vi "Lab Panel V6.00.vi"() -> ()   [LabVIEW 2017] (continued)
                      tunnel: w3847 -> [_ w3860 _ _]
                      tunnel: 0 -> [w3854 w3859 w3864 _]
                      tunnel: w3846 -> [_ _ w3865 _]
                      frame #0 {
                        n2193 = case shown="True" w3855 {
                          tunnel: w3854 -> [w3856 _]
                          frame False {
                            n2194 = local write "Er USB#0"(w3856) -> ()
                          }
                          frame True {
                            n2195 = local read "Er USB#0"() -> (w3858:dbl)
                            n2196 = Increment(x=w3858) -> (x+1=→"Er USB#0":dbl)
                          }
                        }
                      }
                      frame #1 {
                        n2197 = case shown="True" w3860 {
                          tunnel: w3859 -> [w3861 _]
                          frame False {
                            n2198 = local write "Er USB#1"(w3861) -> ()
                          }
                          frame True {
                            n2199 = local read "Er USB#1"() -> (w3863:dbl)
                            n2200 = Increment(x=w3863) -> (x+1=→"Er USB#1":dbl)
                          }
                        }
                      }
                      frame #2 {
                        n2201 = case shown="True" w3865 {
                          tunnel: w3864 -> [w3866 _]
                          frame False {
                            n2202 = local write "Er USB#2"(w3866) -> ()
                          }
                          frame True {
                            n2203 = local read "Er USB#2"() -> (w3868:dbl)
                            n2204 = Increment(x=w3868) -> (x+1=→"Er USB#2":dbl)
                          }
                        }
                      }
                      frame #3 {
                        w3874 = 10
                        n2205 = local read "Er USB#2"() -> (w3875:dbl)
                        n2206 = local read "Er USB#0"() -> (w3877:dbl)
                        n2207 = local read "Er USB#1"() -> (w3876:dbl)
                        n2208 = Greater Or Equal?(x=w3877, y=w3874) -> (x >= y?=w3872:bool)
                        n2209 = Greater Or Equal?(x=w3876, y=w3874) -> (x >= y?=w3871:bool)
                        n2210 = Greater Or Equal?(x=w3875, y=w3874) -> (x >= y?=w3870:bool)
                        n2211 = Or(x=w3872, y=w3871) -> (x .or. y?=w3873:bool)
                        n2212 = Or(x=w3873, y=w3870) -> (x .or. y?=→"Analog error":bool)
                      }
                    }
                  }
                  frame #1 {
                    # "display graph data on ADM page"
                    n2213 = local write "AI loop time"(w3878) -> ()
                    n2214 = local write "AI"(TRUE) -> ()
                    n2215 = Index Array(array=w3899, index=6) -> (element=→"LAB04-1 (GRAPH)":dynamicdata)
                    n2216 = Index Array(array=w3899, index=7) -> (element=→"LAB04-2 (GRAPH)":dynamicdata)
                    n2217 = Index Array(array=w3899, index=9) -> (element=→"LAB05-2 (GRAPH)":dynamicdata)
                    n2218 = Index Array(array=w3899, index=8) -> (element=→"LAB05-1 (GRAPH)":dynamicdata)
                    n2219 = Index Array(array=w3899, index=5) -> (element=→"LAB03-2 (GRAPH)":dynamicdata)
                    n2220 = Index Array(array=w3899, index=0) -> (element=→"LAB01-1 (GRAPH)":dynamicdata)
                    n2221 = Index Array(array=w3899, index=1) -> (element=→"LAB01-2 (GRAPH)":dynamicdata)
                    n2222 = Index Array(array=w3899, index=2) -> (element=→"LAB02-1 (GRAPH)":dynamicdata)
                    n2223 = Index Array(array=w3899, index=3) -> (element=→"LAB02-2 (GRAPH)":dynamicdata)
                    n2224 = Index Array(array=w3899, index=4) -> (element=→"LAB03-1 (GRAPH)":dynamicdata)
                  }
                  frame #2 {
                    n2225 = case shown="False" w3931 {
                      tunnel: [w3933 w3934] -> w3929
                      tunnel: w3930 -> [_ w3934]
                      frame False {
                        n2226 = local read "CAL LAB01"() -> (w3933:T15)
                      }
                      frame True {
                      }
                    }
                    n2227 = Unbundle By Name(w3932) -> ("OFF amps"=w3928:dbl, "VOLTS"=w3927:dbl, "PF"=w3926:dbl, "OFF amps"=w3925:dbl, "VOLTS"=w3924:dbl, "PF"=w3923:dbl)
                    n2228 = Unbundle By Name(w3929) -> ("1  (A) cal"=w3922:dbl, "1 (V) cal"=w3921:dbl, "1 (PF) cal"=w3920:dbl, "2 (A) cal"=w3919:dbl, "2 (V) cal"=w3918:dbl, "2 (PF) cal"=w3917:dbl)  [unwired: 4 out]
                    n2229 = Multiply(x=w3928, y=w3922) -> (x*y=w3912:dbl)
                    n2230 = Multiply(x=w3927, y=w3921) -> (x*y=w3911:dbl)
                    n2231 = Multiply(x=w3926, y=w3920) -> (x*y=w3906:dbl)
                    n2232 = Multiply(x=w3925, y=w3919) -> (x*y=w3909:dbl)
                    n2233 = Multiply(x=w3924, y=w3918) -> (x*y=w3908:dbl)
                    n2234 = Multiply(x=w3923, y=w3917) -> (x*y=w3902:dbl)
                    n2235 = local read "SIG LAB01-2"() -> (w3915:T2)
                    n2236 = call "Check for valid PF.vi"("PF In"=w3906, "VOLTS"=w3911, "Current"=w3912) -> ("PF Out"=w3904:dbl, "V Out"=w3905:dbl, "I Out"=w3910:dbl)  [unwired: 6 in]
                    n2237 = call "Check for valid PF.vi"("PF In"=w3902, "VOLTS"=w3908, "Current"=w3909) -> ("PF Out"=w3901:dbl, "V Out"=w3903:dbl, "I Out"=w3907:dbl)  [unwired: 6 in]
                    n2238 = local read "SIG LAB01-1"() -> (w3916:T2)
                    n2239 = Bundle By Name(cluster=w3916, "AMPS"=w3910, "VOLTS"=w3905, "PF"=w3904) -> (w3914:T2)
                    n2240 = Bundle By Name(cluster=w3915, "AMPS"=w3907, "VOLTS"=w3903, "PF"=w3901) -> (w3913:T2)
                    n2241 = global write "Global display 1.vi" "SIG LAB01-2"(w3913) -> ()
                    n2242 = global write "Global display 1.vi" "SIG LAB01-1"(w3914) -> ()
                    n2243 = local write "SIG LAB01-2"(w3913) -> ()
                    n2244 = local write "SIG LAB01-1"(w3914) -> ()
                  }
                  frame #3 {
                    n2245 = Unbundle By Name(w3966) -> ("OFF amps"=w3962:dbl, "VOLTS"=w3961:dbl, "PF"=w3960:dbl, "OFF amps"=w3959:dbl, "VOLTS"=w3958:dbl, "PF"=w3957:dbl)
                    n2246 = case shown="True" w3965 {
                      tunnel: [w3967 w3968] -> w3963
                      tunnel: w3964 -> [_ w3968]
                      frame False {
                        n2247 = local read "CAL LAB02"() -> (w3967:T16)
                      }
                      frame True {
                      }
                    }
                    n2248 = Unbundle By Name(w3963) -> ("1  (A) cal"=w3956:dbl, "1 (V) cal"=w3955:dbl, "1 (PF) cal"=w3954:dbl, "2 (A) cal"=w3953:dbl, "2 (V) cal"=w3952:dbl, "2 (PF) cal"=w3951:dbl)  [unwired: 4 out]
                    n2249 = Multiply(x=w3962, y=w3956) -> (x*y=w3946:dbl)
                    n2250 = Multiply(x=w3961, y=w3955) -> (x*y=w3945:dbl)
                    n2251 = Multiply(x=w3960, y=w3954) -> (x*y=w3938:dbl)
                    n2252 = Multiply(x=w3959, y=w3953) -> (x*y=w3943:dbl)
                    n2253 = Multiply(x=w3958, y=w3952) -> (x*y=w3942:dbl)
                    n2254 = Multiply(x=w3957, y=w3951) -> (x*y=w3937:dbl)
                    n2255 = local read "SIG LAB02-1"() -> (w3950:T2)
                    n2256 = local read "SIG LAB02-2"() -> (w3949:T2)
                    n2257 = call "Check for valid PF.vi"("PF In"=w3938, "VOLTS"=w3945, "Current"=w3946) -> ("PF Out"=w3940:dbl, "V Out"=w3939:dbl, "I Out"=w3944:dbl)  [unwired: 6 in]
                    n2258 = call "Check for valid PF.vi"("PF In"=w3937, "VOLTS"=w3942, "Current"=w3943) -> ("PF Out"=w3935:dbl, "V Out"=w3936:dbl, "I Out"=w3941:dbl)  [unwired: 6 in]
                    n2259 = Bundle By Name(cluster=w3950, "AMPS"=w3944, "VOLTS"=w3939, "PF"=w3940) -> (w3948:T2)
                    n2260 = Bundle By Name(cluster=w3949, "AMPS"=w3941, "VOLTS"=w3936, "PF"=w3935) -> (w3947:T2)
                    n2261 = global write "Global display 1.vi" "SIG LAB02-1"(w3948) -> ()
                    n2262 = local write "SIG LAB02-2"(w3947) -> ()
                    n2263 = global write "Global display 1.vi" "SIG LAB02-2"(w3947) -> ()
                    n2264 = local write "SIG LAB02-1"(w3948) -> ()
                  }
                  frame #4 {
                    n2265 = Unbundle By Name(w4000) -> ("OFF amps"=w3996:dbl, "VOLTS"=w3995:dbl, "PF"=w3994:dbl, "OFF amps"=w3993:dbl, "VOLTS"=w3992:dbl, "PF"=w3991:dbl)
                    n2266 = case shown="False" w3999 {
                      tunnel: [w4001 w4002] -> w3997
                      tunnel: w3998 -> [_ w4002]
                      frame False {
                        n2267 = local read "CAL LAB03"() -> (w4001:T15)
                      }
                      frame True {
                      }
                    }
                    n2268 = Unbundle By Name(w3997) -> ("1  (A) cal"=w3990:dbl, "1 (V) cal"=w3989:dbl, "1 (PF) cal"=w3988:dbl, "2 (A) cal"=w3987:dbl, "2 (V) cal"=w3986:dbl, "2 (PF) cal"=w3985:dbl)  [unwired: 4 out]
                    n2269 = Multiply(x=w3996, y=w3990) -> (x*y=w3980:dbl)
                    n2270 = Multiply(x=w3995, y=w3989) -> (x*y=w3979:dbl)
                    n2271 = Multiply(x=w3994, y=w3988) -> (x*y=w3974:dbl)
                    n2272 = Multiply(x=w3993, y=w3987) -> (x*y=w3977:dbl)
                    n2273 = Multiply(x=w3992, y=w3986) -> (x*y=w3976:dbl)
                    n2274 = Multiply(x=w3991, y=w3985) -> (x*y=w3973:dbl)
                    n2275 = local read "SIG LAB03-1"() -> (w3984:T2)
                    n2276 = local read "SIG LAB03-2"() -> (w3983:T2)
                    n2277 = call "Check for valid PF.vi"("PF In"=w3974, "VOLTS"=w3979, "Current"=w3980) -> ("PF Out"=w3969:dbl, "V Out"=w3970:dbl, "I Out"=w3978:dbl)  [unwired: 6 in]
                    n2278 = call "Check for valid PF.vi"("PF In"=w3973, "VOLTS"=w3976, "Current"=w3977) -> ("PF Out"=w3972:dbl, "V Out"=w3971:dbl, "I Out"=w3975:dbl)  [unwired: 6 in]
                    n2279 = Bundle By Name(cluster=w3984, "AMPS"=w3978, "VOLTS"=w3970, "PF"=w3969) -> (w3982:T2)
                    n2280 = Bundle By Name(cluster=w3983, "AMPS"=w3975, "VOLTS"=w3971, "PF"=w3972) -> (w3981:T2)
                    n2281 = global write "Global display 1.vi" "SIG LAB03-1"(w3982) -> ()
                    n2282 = global write "Global display 1.vi" "SIG LAB03-2"(w3981) -> ()
                    n2283 = local write "SIG LAB03-2"(w3981) -> ()
                    n2284 = local write "SIG LAB03-1"(w3982) -> ()
                  }
                  frame #5 {
                    n2285 = case shown="False" w4033 {
                      tunnel: [w4035 w4036] -> w4031
                      tunnel: w4032 -> [_ w4036]
                      frame False {
                        n2286 = local read "CAL LAB04"() -> (w4035:T15)
                      }
                      frame True {
                      }
                    }
                    n2287 = Unbundle By Name(w4034) -> ("OFF amps"=w4030:dbl, "VOLTS"=w4029:dbl, "PF"=w4028:dbl, "OFF amps"=w4027:dbl, "VOLTS"=w4026:dbl, "PF"=w4025:dbl)
                    n2288 = Unbundle By Name(w4031) -> ("1  (A) cal"=w4024:dbl, "1 (V) cal"=w4023:dbl, "1 (PF) cal"=w4022:dbl, "2 (A) cal"=w4021:dbl, "2 (V) cal"=w4020:dbl, "2 (PF) cal"=w4019:dbl)  [unwired: 4 out]
                    n2289 = Multiply(x=w4030, y=w4024) -> (x*y=w4014:dbl)
                    n2290 = Multiply(x=w4029, y=w4023) -> (x*y=w4013:dbl)
                    n2291 = Multiply(x=w4028, y=w4022) -> (x*y=w4004:dbl)
                    n2292 = Multiply(x=w4027, y=w4021) -> (x*y=w4011:dbl)
                    n2293 = Multiply(x=w4026, y=w4020) -> (x*y=w4010:dbl)
                    n2294 = Multiply(x=w4025, y=w4019) -> (x*y=w4003:dbl)
                    n2295 = local read "SIG LAB04-1"() -> (w4018:T2)
                    n2296 = local read "SIG LAB04-2"() -> (w4017:T2)
                    n2297 = call "Check for valid PF.vi"("PF In"=w4004, "VOLTS"=w4013, "Current"=w4014) -> ("PF Out"=w4007:dbl, "V Out"=w4008:dbl, "I Out"=w4012:dbl)  [unwired: 6 in]
                    n2298 = call "Check for valid PF.vi"("PF In"=w4003, "VOLTS"=w4010, "Current"=w4011) -> ("PF Out"=w4005:dbl, "V Out"=w4006:dbl, "I Out"=w4009:dbl)  [unwired: 6 in]
                    n2299 = Bundle By Name(cluster=w4018, "AMPS"=w4012, "VOLTS"=w4008, "PF"=w4007) -> (w4016:T2)
                    n2300 = Bundle By Name(cluster=w4017, "AMPS"=w4009, "VOLTS"=w4006, "PF"=w4005) -> (w4015:T2)
                    n2301 = global write "Global display 1.vi" "SIG LAB04-2"(w4015) -> ()
                    n2302 = global write "Global display 1.vi" "SIG LAB04-1"(w4016) -> ()
                    n2303 = local write "SIG LAB04-2"(w4015) -> ()
                    n2304 = local write "SIG LAB04-1"(w4016) -> ()
                  }
                  frame #6 {
                    n2305 = Unbundle By Name(w4068) -> ("OFF amps"=w4064:dbl, "VOLTS"=w4051:dbl, "PF"=w4063:dbl, "OFF amps"=w4062:dbl, "VOLTS"=w4061:dbl, "PF"=w4060:dbl)
                    n2306 = case shown="False" w4067 {
                      tunnel: [w4069 w4070] -> w4065
                      tunnel: w4066 -> [_ w4070]
                      frame False {
                        n2307 = local read "CAL LAB05"() -> (w4069:T15)
                      }
                      frame True {
                      }
                    }
                    n2308 = Unbundle By Name(w4065) -> ("1  (A) cal"=w4059:dbl, "1 (V) cal"=w4058:dbl, "1 (PF) cal"=w4057:dbl, "2 (A) cal"=w4056:dbl, "2 (V) cal"=w4055:dbl, "2 (PF) cal"=w4054:dbl)  [unwired: 4 out]
                    n2309 = Multiply(x=w4064, y=w4059) -> (x*y=w4048:dbl)
                    n2310 = Multiply(x=w4051, y=w4058) -> (x*y=w4047:dbl)
                    n2311 = Multiply(x=w4063, y=w4057) -> (x*y=w4042:dbl)
                    n2312 = Multiply(x=w4062, y=w4056) -> (x*y=w4045:dbl)
                    n2313 = Multiply(x=w4061, y=w4055) -> (x*y=w4044:dbl)
                    n2314 = Multiply(x=w4060, y=w4054) -> (x*y=w4039:dbl)
                    n2315 = local read "SIG LAB05-1"() -> (w4053:T2)
                    n2316 = local read "SIG LAB05-2"() -> (w4052:T2)
                    n2317 = call "Check for valid PF.vi"("PF In"=w4039, "VOLTS"=w4044, "Current"=w4045) -> ("PF Out"=w4038:dbl, "V Out"=w4037:dbl, "I Out"=w4043:dbl)  [unwired: 6 in]
                    n2318 = call "Check for valid PF.vi"("PF In"=w4042, "VOLTS"=w4047, "Current"=w4048) -> ("PF Out"=w4041:dbl, "V Out"=w4040:dbl, "I Out"=w4046:dbl)  [unwired: 6 in]
                    n2319 = Bundle By Name(cluster=w4053, "AMPS"=w4046, "VOLTS"=w4040, "PF"=w4041) -> (w4050:T2)
                    n2320 = Bundle By Name(cluster=w4052, "AMPS"=w4043, "VOLTS"=w4037, "PF"=w4038) -> (w4049:T2)
                    n2321 = global write "Global display 1.vi" "SIG LAB05-1"(w4050) -> ()
                    n2322 = global write "Global display 1.vi" "SIG LAB05-2"(w4049) -> ()
                    n2323 = local write "SIG LAB05-2"(w4049) -> ()
                    n2324 = local write "SIG LAB05-1"(w4050) -> ()
                  }
                  frame #7 {
                    n2325 = case shown="False" w4071 {
                      tunnel: w4073 -> [w4078 _]
                      tunnel: w4072 -> [w4077 _]
                      frame False {
                        # "update ambient referance temperature"
                        n2326 = case shown="False" w4078 {
                          tunnel: [w4080 100.0] -> w4079
                          frame False {
                            n2327 = local read "TEMP REF cal"() -> (w4080:dbl)
                          }
                          frame True {
                          }
                        }
                        n2328 = disable-structure shown="Disabled" {
                          frame Disabled {
                            n2329 = local read "Temp read loop"() -> ()  [unwired: 1 out]
                          }
                          frame Enabled {
                          }
                        }
                        n2330 = Multiply(x=w4079, y=w4077) -> (x*y=w4076:dbl)
                        n2331 = Subtract(x=w4076, y=272) -> (x-y=w4074:dbl)
                        "Amb Temp" <- w4074
                        n2332 = local write "Ref deg C"(w4074) -> ()
                        "deg C (volts)" <- w4077
                      }
                      frame True {
                      }
                    }
                  }
                }
              }
            }
          }
          frame #14 {
            # "save test data to file during testing"
            n2333 = local read "on loops"() -> (w4101:dbl)
            n2334 = Get Date/Time In Seconds() -> (seconds since 1Jan1904=w4082:timestamp)
            "File Time Stamp" <- w4082
            n2335 = local read "jig cycle"() -> (w4098:dbl)
            n2336 = Format Date/Time String(time format string (%c)="%H:%M%:%S", seconds (now)=w4082) -> (date/time string=w4086:string)  [unwired: 1 in]
            n2337 = Add(x=w4101, y=4) -> (x+y=w4099:dbl)
            n2338 = Build Array(w4086) -> (w4085:string[])
            n2339 = Equal?(x=w4098, y=3) -> (x = y?=w4084:bool)
            n2340 = Equal?(x=w4098, y=w4099) -> (x = y?=w4083:bool)
            n2341 = stacked-sequence {
              tunnel: w4097 -> [w4107 _ _ _ _ _ _ _ _ _]
              tunnel: w4096 -> [_ w4183 _ _ _ _ _ _ _ _]
              tunnel: w4095 -> [_ _ w4263 _ _ _ _ _ _ _]
              tunnel: w4094 -> [_ _ _ w4343 _ _ _ _ _ _]
              tunnel: w4093 -> [_ _ _ _ w4423 _ _ _ _ _]
              tunnel: w4092 -> [_ _ _ _ _ w4503 _ _ _ _]
              tunnel: w4091 -> [_ _ _ _ _ _ w4583 _ _ _]
              tunnel: w4090 -> [_ _ _ _ _ _ _ w4663 _ _]
              tunnel: w4089 -> [_ _ _ _ _ _ _ _ w4743 _]
              tunnel: w4088 -> [_ _ _ _ _ _ _ _ _ w4823]
              tunnel: w4085 -> [w4106 w4187 w4267 w4347 w4427 w4507 w4587 w4667 w4747 w4827]
              tunnel: w4084 -> [w4105 w4186 w4266 w4346 w4426 w4506 w4586 w4666 w4746 w4826]
              tunnel: w4083 -> [w4104 w4185 w4265 w4345 w4425 w4505 w4585 w4665 w4745 w4825]
              tunnel: w4082 -> [w4103 w4184 w4264 w4344 w4424 w4504 w4584 w4664 w4744 w4824]
              frame #0 {
                n2342 = case shown="True" w4107 {
                  tunnel: w4106 -> [_ w4112]
                  tunnel: w4105 -> [_ w4111]
                  tunnel: w4104 -> [_ w4109]
                  tunnel: w4103 -> [_ w4108]
                  frame False {
                  }
                  frame True {
                    n2343 = local read "SIG LAB01-1"() -> (w4114:T2)
                    n2344 = local read "ON L01-1"() -> (w4110:cluster{"amps":dbl, "volts":dbl, "pf":dbl})
                    n2345 = local read "DISP LAB01-1"() -> (w4113:T4)
                    n2346 = Unbundle(w4114) -> ("AMPS"=w4120:dbl, "VOLTS"=w4118:dbl, "PF"=w4117:dbl, "Tmp Live"=w4116:dbl, "Tmp Neut"=w4119:dbl)
                    n2347 = Unbundle(w4113) -> ("CYCLE"=w4115:dbl)  [unwired: 2 out]
                    n2348 = stacked-sequence {
                      tunnel: w4120 -> [w4124 w4143]
                      tunnel: w4119 -> [_ w4142]
                      tunnel: w4118 -> [w4123 w4141]
                      tunnel: w4117 -> [w4122 w4140]
                      tunnel: w4116 -> [_ w4139]
                      tunnel: w4115 -> [_ w4138]
                      tunnel: w4112 -> [_ w4137]
                      tunnel: w4111 -> [w4125 _]
                      tunnel: w4110 -> [w4121 w4135]
                      tunnel: w4109 -> [_ w4136]
                      tunnel: w4108 -> [_ w4131]
                      frame #0 {
                        n2349 = case shown="True" w4125 {
                          tunnel: w4124 -> [_ w4130]
                          tunnel: w4123 -> [_ w4129]
                          tunnel: w4122 -> [_ w4128]
                          tunnel: w4121 -> [_ w4126]
                          frame False {
                          }
                          frame True {
                            n2350 = Bundle(cluster=w4126, "amps"=w4130, "volts"=w4129, "pf"=w4128) -> (w4127:cluster{"amps":dbl, "volts":dbl, "pf":dbl})
                            n2351 = local write "ON L01-1"(w4127) -> ()
                          }
                        }
                      }
                      frame #1 {
                        n2352 = Unbundle(w4135) -> ("amps"=w4134:dbl, "volts"=w4133:dbl, "pf"=w4132:dbl)
                        n2353 = case shown="True" w4136 {
                          tunnel: w4143 -> [_ w4144]
                          tunnel: w4142 -> [_ w4182]
                          tunnel: w4141 -> [_ _]
                          tunnel: w4140 -> [_ _]
                          tunnel: w4139 -> [_ w4181]
                          tunnel: w4138 -> [_ w4180]
                          tunnel: w4137 -> [_ w4148]
                          tunnel: w4134 -> [_ w4145]
                          tunnel: w4133 -> [_ w4177]
                          tunnel: w4132 -> [_ w4176]
                          tunnel: w4131 -> [_ w4146]
                          frame False {
                          }
                          frame True {
                            n2354 = local read "TDMS LAB01-1"() -> (w4179:refnum<k34>)
                            n2355 = Build Array(w4177) -> (w4173:dbl[])
                            n2356 = Build Array(w4176) -> (w4172:dbl[])
                            n2357 = Build Array(w4181) -> (w4171:dbl[])
                            n2358 = Build Array(w4182) -> (w4170:dbl[])
                            n2359 = Build Array(w4145) -> (w4175:dbl[])
                            n2360 = Build Array(w4144) -> (w4174:dbl[])
                            n2361 = Build Array(w4180) -> (w4169:dbl[])
                            n2362 = Build Array("AMPS ON", "AMPS OFF", "VOLTS", "PF", "TEMP Live", "TEMP Neut", "CYCLE") -> (w4153:string[])
                            n2363 = Bundle By Name("Y"=w4175, "t0"=w4146) -> (w4168:waveform(dbl))  [unwired: 1 in]
                            n2364 = Bundle By Name("Y"=w4174, "t0"=w4146) -> (w4167:waveform(dbl))  [unwired: 1 in]
                            n2365 = Bundle By Name("Y"=w4173, "t0"=w4146) -> (w4166:waveform(dbl))  [unwired: 1 in]
                            n2366 = Bundle By Name("Y"=w4172, "t0"=w4146) -> (w4165:waveform(dbl))  [unwired: 1 in]
                            n2367 = Bundle By Name("Y"=w4171, "t0"=w4146) -> (w4164:waveform(dbl))  [unwired: 1 in]
                            n2368 = Bundle By Name("Y"=w4170, "t0"=w4146) -> (w4163:waveform(dbl))  [unwired: 1 in]
                            n2369 = Bundle By Name("Y"=w4169, "t0"=w4146) -> (w4162:waveform(dbl))  [unwired: 1 in]
                            n2370 = Build Array(w4168, w4167, w4166, w4165, w4164, w4163, w4162) -> (w4161:waveform(dbl)[])
                            n2371 = TDMS Write(0:w4179, 5:"TEST VALUES", 7:w4153, 9:w4161) -> (4:w4152:refnum<k34>, 6:w4151:string, 15:w4150:errorcluster)  [unwired: 2 in, 1 out]
                            n2372 = TDMS Write(0:w4152, 5:w4151, 7:"TIME", 9:w4148, 11:w4150) -> (15:w4147:errorcluster)  [unwired: 1 in, 3 out]
                            n2373 = local write "data file error"(w4147) -> ()
                          }
                        }
                      }
                    }
                  }
                }
              }
              frame #1 {
                n2374 = case shown="True" w4183 {
                  tunnel: w4187 -> [_ w4192]
                  tunnel: w4186 -> [_ w4191]
                  tunnel: w4185 -> [_ w4189]
                  tunnel: w4184 -> [_ w4188]
                  frame False {
                  }
                  frame True {
                    n2375 = local read "DISP LAB01-2"() -> (w4193:T4)
                    n2376 = local read "SIG LAB01-2"() -> (w4194:T2)
                    n2377 = local read "ON L01-2"() -> (w4190:cluster{"amps":dbl, "volts":dbl, "pf":dbl})
                    n2378 = Unbundle(w4194) -> ("AMPS"=w4200:dbl, "VOLTS"=w4198:dbl, "PF"=w4197:dbl, "Tmp Live"=w4196:dbl, "Tmp Neut"=w4199:dbl)
                    n2379 = Unbundle(w4193) -> ("CYCLE"=w4195:dbl)  [unwired: 2 out]
                    n2380 = stacked-sequence {
                      tunnel: w4200 -> [w4204 w4223]
                      tunnel: w4199 -> [_ w4222]
                      tunnel: w4198 -> [w4203 w4221]
                      tunnel: w4197 -> [w4202 w4220]
                      tunnel: w4196 -> [_ w4219]
                      tunnel: w4195 -> [_ w4218]
                      tunnel: w4192 -> [_ w4217]
                      tunnel: w4191 -> [w4205 _]
                      tunnel: w4190 -> [w4201 w4215]
                      tunnel: w4189 -> [_ w4216]
                      tunnel: w4188 -> [_ w4211]
                      frame #0 {
                        n2381 = case shown="True" w4205 {
                          tunnel: w4204 -> [_ w4210]
                          tunnel: w4203 -> [_ w4209]
                          tunnel: w4202 -> [_ w4208]
                          tunnel: w4201 -> [_ w4206]
                          frame False {
                          }
                          frame True {
                            n2382 = Bundle(cluster=w4206, "amps"=w4210, "volts"=w4209, "pf"=w4208) -> (w4207:cluster{"amps":dbl, "volts":dbl, "pf":dbl})
                            n2383 = local write "ON L01-2"(w4207) -> ()
                          }
                        }
                      }
                      frame #1 {
                        n2384 = Unbundle(w4215) -> ("amps"=w4214:dbl, "volts"=w4213:dbl, "pf"=w4212:dbl)
                        n2385 = case shown="True" w4216 {
                          tunnel: w4223 -> [_ w4255]
                          tunnel: w4222 -> [_ w4262]
                          tunnel: w4221 -> [_ _]
                          tunnel: w4220 -> [_ _]
                          tunnel: w4219 -> [_ w4261]
                          tunnel: w4218 -> [_ w4260]
                          tunnel: w4217 -> [_ w4225]
                          tunnel: w4214 -> [_ w4257]
                          tunnel: w4213 -> [_ w4256]
                          tunnel: w4212 -> [_ w4254]
                          tunnel: w4211 -> [_ w4246]
                          frame False {
                          }
                          frame True {
                            n2386 = local read "TDMS LAB01-2"() -> (w4259:refnum<k34>)
                            n2387 = Build Array(w4256) -> (w4251:dbl[])
                            n2388 = Build Array(w4254) -> (w4250:dbl[])
                            n2389 = Build Array(w4261) -> (w4249:dbl[])
                            n2390 = Build Array(w4262) -> (w4248:dbl[])
                            n2391 = Build Array(w4257) -> (w4253:dbl[])
                            n2392 = Build Array(w4255) -> (w4252:dbl[])
                            n2393 = Build Array(w4260) -> (w4247:dbl[])
                            n2394 = Build Array("AMPS ON", "AMPS OFF", "VOLTS", "PF", "TEMP Live", "TEMP Neut", "CYCLE") -> (w4230:string[])
                            n2395 = Bundle By Name("Y"=w4253, "t0"=w4246) -> (w4245:waveform(dbl))  [unwired: 1 in]
                            n2396 = Bundle By Name("Y"=w4252, "t0"=w4246) -> (w4244:waveform(dbl))  [unwired: 1 in]
                            n2397 = Bundle By Name("Y"=w4251, "t0"=w4246) -> (w4243:waveform(dbl))  [unwired: 1 in]
                            n2398 = Bundle By Name("Y"=w4250, "t0"=w4246) -> (w4242:waveform(dbl))  [unwired: 1 in]
                            n2399 = Bundle By Name("Y"=w4249, "t0"=w4246) -> (w4241:waveform(dbl))  [unwired: 1 in]
                            n2400 = Bundle By Name("Y"=w4248, "t0"=w4246) -> (w4240:waveform(dbl))  [unwired: 1 in]
                            n2401 = Bundle By Name("Y"=w4247, "t0"=w4246) -> (w4239:waveform(dbl))  [unwired: 1 in]
                            n2402 = Build Array(w4245, w4244, w4243, w4242, w4241, w4240, w4239) -> (w4238:waveform(dbl)[])
                            n2403 = TDMS Write(0:w4259, 5:"TEST VALUES", 7:w4230, 9:w4238) -> (4:w4229:refnum<k34>, 6:w4228:string, 15:w4227:errorcluster)  [unwired: 2 in, 1 out]
                            n2404 = TDMS Write(0:w4229, 5:w4228, 7:"TIME", 9:w4225, 11:w4227) -> (15:w4224:errorcluster)  [unwired: 1 in, 3 out]
                            n2405 = local write "data file error"(w4224) -> ()
                          }
                        }
                      }
                    }
                  }
                }
              }
              frame #2 {
                n2406 = case shown="True" w4263 {
                  tunnel: w4267 -> [_ w4272]
                  tunnel: w4266 -> [_ w4271]
                  tunnel: w4265 -> [_ w4269]
                  tunnel: w4264 -> [_ w4268]
                  frame False {
                  }
                  frame True {
                    n2407 = local read "DISP LAB02-1"() -> (w4273:T4)
                    n2408 = local read "SIG LAB02-1"() -> (w4274:T2)
                    n2409 = local read "ON L02-1"() -> (w4270:cluster{"amps":dbl, "volts":dbl, "pf":dbl})
                    n2410 = Unbundle(w4274) -> ("AMPS"=w4280:dbl, "VOLTS"=w4278:dbl, "PF"=w4277:dbl, "Tmp Live"=w4276:dbl, "Tmp Neut"=w4279:dbl)
                    n2411 = Unbundle(w4273) -> ("CYCLE"=w4275:dbl)  [unwired: 2 out]
                    n2412 = stacked-sequence {
                      tunnel: w4280 -> [w4284 w4303]
                      tunnel: w4279 -> [_ w4302]
                      tunnel: w4278 -> [w4283 w4301]
                      tunnel: w4277 -> [w4282 w4300]
                      tunnel: w4276 -> [_ w4299]
                      tunnel: w4275 -> [_ w4298]
                      tunnel: w4272 -> [_ w4297]
                      tunnel: w4271 -> [w4285 _]
                      tunnel: w4270 -> [w4281 w4295]
                      tunnel: w4269 -> [_ w4296]
                      tunnel: w4268 -> [_ w4291]
                      frame #0 {
                        n2413 = case shown="True" w4285 {
                          tunnel: w4284 -> [_ w4290]
                          tunnel: w4283 -> [_ w4289]
                          tunnel: w4282 -> [_ w4288]
                          tunnel: w4281 -> [_ w4286]
                          frame False {
                          }
                          frame True {
                            n2414 = Bundle(cluster=w4286, "amps"=w4290, "volts"=w4289, "pf"=w4288) -> (w4287:cluster{"amps":dbl, "volts":dbl, "pf":dbl})
                            n2415 = local write "ON L02-1"(w4287) -> ()
                          }
                        }
                      }
                      frame #1 {
                        n2416 = Unbundle(w4295) -> ("amps"=w4294:dbl, "volts"=w4293:dbl, "pf"=w4292:dbl)
                        n2417 = case shown="True" w4296 {
                          tunnel: w4303 -> [_ w4335]
                          tunnel: w4302 -> [_ w4342]
                          tunnel: w4301 -> [_ _]
                          tunnel: w4300 -> [_ _]
                          tunnel: w4299 -> [_ w4341]
                          tunnel: w4298 -> [_ w4340]
                          tunnel: w4297 -> [_ w4305]
                          tunnel: w4294 -> [_ w4337]
                          tunnel: w4293 -> [_ w4336]
                          tunnel: w4292 -> [_ w4334]
                          tunnel: w4291 -> [_ w4326]
                          frame False {
                          }
                          frame True {
                            n2418 = local read "TDMS LAB02-1"() -> (w4339:refnum<k34>)
                            n2419 = Build Array(w4336) -> (w4331:dbl[])
                            n2420 = Build Array(w4334) -> (w4330:dbl[])
                            n2421 = Build Array(w4341) -> (w4329:dbl[])
                            n2422 = Build Array(w4342) -> (w4328:dbl[])
                            n2423 = Build Array(w4337) -> (w4333:dbl[])
                            n2424 = Build Array(w4335) -> (w4332:dbl[])
                            n2425 = Build Array(w4340) -> (w4327:dbl[])
                            n2426 = Build Array("AMPS ON", "AMPS OFF", "VOLTS", "PF", "TEMP Live", "TEMP Neut", "CYCLE") -> (w4310:string[])
                            n2427 = Bundle By Name("Y"=w4333, "t0"=w4326) -> (w4325:waveform(dbl))  [unwired: 1 in]
                            n2428 = Bundle By Name("Y"=w4332, "t0"=w4326) -> (w4324:waveform(dbl))  [unwired: 1 in]
                            n2429 = Bundle By Name("Y"=w4331, "t0"=w4326) -> (w4323:waveform(dbl))  [unwired: 1 in]
                            n2430 = Bundle By Name("Y"=w4330, "t0"=w4326) -> (w4322:waveform(dbl))  [unwired: 1 in]
                            n2431 = Bundle By Name("Y"=w4329, "t0"=w4326) -> (w4321:waveform(dbl))  [unwired: 1 in]
                            n2432 = Bundle By Name("Y"=w4328, "t0"=w4326) -> (w4320:waveform(dbl))  [unwired: 1 in]
                            n2433 = Bundle By Name("Y"=w4327, "t0"=w4326) -> (w4319:waveform(dbl))  [unwired: 1 in]
                            n2434 = Build Array(w4325, w4324, w4323, w4322, w4321, w4320, w4319) -> (w4318:waveform(dbl)[])
                            n2435 = TDMS Write(0:w4339, 5:"TEST VALUES", 7:w4310, 9:w4318) -> (4:w4309:refnum<k34>, 6:w4308:string, 15:w4307:errorcluster)  [unwired: 2 in, 1 out]
                            n2436 = TDMS Write(0:w4309, 5:w4308, 7:"TIME", 9:w4305, 11:w4307) -> (15:w4304:errorcluster)  [unwired: 1 in, 3 out]
                            n2437 = local write "data file error"(w4304) -> ()
                          }
                        }
                      }
                    }
                  }
                }
              }
              frame #3 {
                n2438 = case shown="True" w4343 {
                  tunnel: w4347 -> [_ w4352]
                  tunnel: w4346 -> [_ w4351]
                  tunnel: w4345 -> [_ w4349]
                  tunnel: w4344 -> [_ w4348]
                  frame False {
                  }
                  frame True {
                    n2439 = local read "DISP LAB02-2"() -> (w4353:T4)
                    n2440 = local read "SIG LAB02-2"() -> (w4354:T2)
                    n2441 = local read "ON L02-2"() -> (w4350:cluster{"amps":dbl, "volts":dbl, "pf":dbl})
                    n2442 = Unbundle(w4354) -> ("AMPS"=w4360:dbl, "VOLTS"=w4358:dbl, "PF"=w4357:dbl, "Tmp Live"=w4356:dbl, "Tmp Neut"=w4359:dbl)
                    n2443 = Unbundle(w4353) -> ("CYCLE"=w4355:dbl)  [unwired: 2 out]
                    n2444 = stacked-sequence {
                      tunnel: w4360 -> [w4364 w4383]
                      tunnel: w4359 -> [_ w4382]
                      tunnel: w4358 -> [w4363 w4381]
                      tunnel: w4357 -> [w4362 w4380]
                      tunnel: w4356 -> [_ w4379]
                      tunnel: w4355 -> [_ w4378]
                      tunnel: w4352 -> [_ w4377]
                      tunnel: w4351 -> [w4365 _]
                      tunnel: w4350 -> [w4361 w4375]
                      tunnel: w4349 -> [_ w4376]
                      tunnel: w4348 -> [_ w4371]
                      frame #0 {
                        n2445 = case shown="True" w4365 {
                          tunnel: w4364 -> [_ w4370]
                          tunnel: w4363 -> [_ w4369]
                          tunnel: w4362 -> [_ w4368]
                          tunnel: w4361 -> [_ w4366]
                          frame False {
                          }
                          frame True {
                            n2446 = Bundle(cluster=w4366, "amps"=w4370, "volts"=w4369, "pf"=w4368) -> (w4367:cluster{"amps":dbl, "volts":dbl, "pf":dbl})
                            n2447 = local write "ON L02-2"(w4367) -> ()
                          }
                        }
                      }
                      frame #1 {
                        n2448 = Unbundle(w4375) -> ("amps"=w4374:dbl, "volts"=w4373:dbl, "pf"=w4372:dbl)
                        n2449 = case shown="True" w4376 {
                          tunnel: w4383 -> [_ w4415]
                          tunnel: w4382 -> [_ w4422]
                          tunnel: w4381 -> [_ _]
                          tunnel: w4380 -> [_ _]
                          tunnel: w4379 -> [_ w4421]
                          tunnel: w4378 -> [_ w4420]
                          tunnel: w4377 -> [_ w4385]
                          tunnel: w4374 -> [_ w4417]
                          tunnel: w4373 -> [_ w4416]
                          tunnel: w4372 -> [_ w4414]
                          tunnel: w4371 -> [_ w4406]
                          frame False {
                          }
                          frame True {
                            n2450 = local read "TDMS LAB02-2"() -> (w4419:refnum<k34>)
                            n2451 = Build Array(w4416) -> (w4411:dbl[])
                            n2452 = Build Array(w4414) -> (w4410:dbl[])
                            n2453 = Build Array(w4421) -> (w4409:dbl[])
                            n2454 = Build Array(w4422) -> (w4408:dbl[])
                            n2455 = Build Array(w4417) -> (w4413:dbl[])
                            n2456 = Build Array(w4415) -> (w4412:dbl[])
                            n2457 = Build Array(w4420) -> (w4407:dbl[])
                            n2458 = Build Array("AMPS ON", "AMPS OFF", "VOLTS", "PF", "TEMP Live", "TEMP Neut", "CYCLE") -> (w4390:string[])
                            n2459 = Bundle By Name("Y"=w4413, "t0"=w4406) -> (w4405:waveform(dbl))  [unwired: 1 in]
                            n2460 = Bundle By Name("Y"=w4412, "t0"=w4406) -> (w4404:waveform(dbl))  [unwired: 1 in]
                            n2461 = Bundle By Name("Y"=w4411, "t0"=w4406) -> (w4403:waveform(dbl))  [unwired: 1 in]
                            n2462 = Bundle By Name("Y"=w4410, "t0"=w4406) -> (w4402:waveform(dbl))  [unwired: 1 in]
                            n2463 = Bundle By Name("Y"=w4409, "t0"=w4406) -> (w4401:waveform(dbl))  [unwired: 1 in]
                            n2464 = Bundle By Name("Y"=w4408, "t0"=w4406) -> (w4400:waveform(dbl))  [unwired: 1 in]
                            n2465 = Bundle By Name("Y"=w4407, "t0"=w4406) -> (w4399:waveform(dbl))  [unwired: 1 in]
                            n2466 = Build Array(w4405, w4404, w4403, w4402, w4401, w4400, w4399) -> (w4398:waveform(dbl)[])
                            n2467 = TDMS Write(0:w4419, 5:"TEST VALUES", 7:w4390, 9:w4398) -> (4:w4389:refnum<k34>, 6:w4388:string, 15:w4387:errorcluster)  [unwired: 2 in, 1 out]
                            n2468 = TDMS Write(0:w4389, 5:w4388, 7:"TIME", 9:w4385, 11:w4387) -> (15:w4384:errorcluster)  [unwired: 1 in, 3 out]
                            n2469 = local write "data file error"(w4384) -> ()
                          }
                        }
                      }
                    }
                  }
                }
              }
              frame #4 {
                n2470 = case shown="True" w4423 {
                  tunnel: w4427 -> [_ w4432]
                  tunnel: w4426 -> [_ w4431]
                  tunnel: w4425 -> [_ w4429]
                  tunnel: w4424 -> [_ w4428]
                  frame False {
                  }
                  frame True {
                    n2471 = local read "DISP LAB03-1"() -> (w4433:T4)
                    n2472 = local read "SIG LAB03-1"() -> (w4434:T2)
                    n2473 = local read "ON L03-1"() -> (w4430:cluster{"amps":dbl, "volts":dbl, "pf":dbl})
                    n2474 = Unbundle(w4434) -> ("AMPS"=w4440:dbl, "VOLTS"=w4438:dbl, "PF"=w4437:dbl, "Tmp Live"=w4436:dbl, "Tmp Neut"=w4439:dbl)
                    n2475 = Unbundle(w4433) -> ("CYCLE"=w4435:dbl)  [unwired: 2 out]
                    n2476 = stacked-sequence {
                      tunnel: w4440 -> [w4444 w4463]
                      tunnel: w4439 -> [_ w4462]
                      tunnel: w4438 -> [w4443 w4461]
                      tunnel: w4437 -> [w4442 w4460]
                      tunnel: w4436 -> [_ w4459]
                      tunnel: w4435 -> [_ w4458]
                      tunnel: w4432 -> [_ w4457]
                      tunnel: w4431 -> [w4445 _]
                      tunnel: w4430 -> [w4441 w4455]
                      tunnel: w4429 -> [_ w4456]
                      tunnel: w4428 -> [_ w4451]
                      frame #0 {
                        n2477 = case shown="True" w4445 {
                          tunnel: w4444 -> [_ w4450]
                          tunnel: w4443 -> [_ w4449]
                          tunnel: w4442 -> [_ w4448]
                          tunnel: w4441 -> [_ w4446]
                          frame False {
                          }
                          frame True {
                            n2478 = Bundle(cluster=w4446, "amps"=w4450, "volts"=w4449, "pf"=w4448) -> (w4447:cluster{"amps":dbl, "volts":dbl, "pf":dbl})
                            n2479 = local write "ON L03-1"(w4447) -> ()
                          }
                        }
                      }
                      frame #1 {
                        n2480 = Unbundle(w4455) -> ("amps"=w4454:dbl, "volts"=w4453:dbl, "pf"=w4452:dbl)
                        n2481 = case shown="True" w4456 {
                          tunnel: w4463 -> [_ w4495]
                          tunnel: w4462 -> [_ w4502]
                          tunnel: w4461 -> [_ _]
                          tunnel: w4460 -> [_ _]
                          tunnel: w4459 -> [_ w4501]
                          tunnel: w4458 -> [_ w4500]
                          tunnel: w4457 -> [_ w4465]
                          tunnel: w4454 -> [_ w4497]
                          tunnel: w4453 -> [_ w4496]
                          tunnel: w4452 -> [_ w4494]
                          tunnel: w4451 -> [_ w4486]
                          frame False {
                          }
                          frame True {
                            n2482 = local read "TDMS LAB03-1"() -> (w4499:refnum<k34>)
                            n2483 = Build Array(w4496) -> (w4491:dbl[])
                            n2484 = Build Array(w4494) -> (w4490:dbl[])
                            n2485 = Build Array(w4501) -> (w4489:dbl[])
                            n2486 = Build Array(w4502) -> (w4488:dbl[])
                            n2487 = Build Array(w4497) -> (w4493:dbl[])
                            n2488 = Build Array(w4495) -> (w4492:dbl[])
                            n2489 = Build Array(w4500) -> (w4487:dbl[])
                            n2490 = Build Array("AMPS ON", "AMPS OFF", "VOLTS", "PF", "TEMP Live", "TEMP Neut", "CYCLE") -> (w4470:string[])
                            n2491 = Bundle By Name("Y"=w4493, "t0"=w4486) -> (w4485:waveform(dbl))  [unwired: 1 in]
                            n2492 = Bundle By Name("Y"=w4492, "t0"=w4486) -> (w4484:waveform(dbl))  [unwired: 1 in]
                            n2493 = Bundle By Name("Y"=w4491, "t0"=w4486) -> (w4483:waveform(dbl))  [unwired: 1 in]
                            n2494 = Bundle By Name("Y"=w4490, "t0"=w4486) -> (w4482:waveform(dbl))  [unwired: 1 in]
                            n2495 = Bundle By Name("Y"=w4489, "t0"=w4486) -> (w4481:waveform(dbl))  [unwired: 1 in]
                            n2496 = Bundle By Name("Y"=w4488, "t0"=w4486) -> (w4480:waveform(dbl))  [unwired: 1 in]
                            n2497 = Bundle By Name("Y"=w4487, "t0"=w4486) -> (w4479:waveform(dbl))  [unwired: 1 in]
                            n2498 = Build Array(w4485, w4484, w4483, w4482, w4481, w4480, w4479) -> (w4478:waveform(dbl)[])
                            n2499 = TDMS Write(0:w4499, 5:"TEST VALUES", 7:w4470, 9:w4478) -> (4:w4469:refnum<k34>, 6:w4468:string, 15:w4467:errorcluster)  [unwired: 2 in, 1 out]
                            n2500 = TDMS Write(0:w4469, 5:w4468, 7:"TIME", 9:w4465, 11:w4467) -> (15:w4464:errorcluster)  [unwired: 1 in, 3 out]
                            n2501 = local write "data file error"(w4464) -> ()
                          }
                        }
                      }
                    }
                  }
                }
              }
              frame #5 {
                n2502 = case shown="True" w4503 {
                  tunnel: w4507 -> [_ w4512]
                  tunnel: w4506 -> [_ w4511]
                  tunnel: w4505 -> [_ w4509]
                  tunnel: w4504 -> [_ w4508]
                  frame False {
                  }
                  frame True {
                    n2503 = local read "DISP LAB03-2"() -> (w4513:T4)
                    n2504 = local read "SIG LAB03-2"() -> (w4514:T2)
                    n2505 = local read "ON L03-2"() -> (w4510:cluster{"amps":dbl, "volts":dbl, "pf":dbl})
                    n2506 = Unbundle(w4514) -> ("AMPS"=w4520:dbl, "VOLTS"=w4518:dbl, "PF"=w4517:dbl, "Tmp Live"=w4516:dbl, "Tmp Neut"=w4519:dbl)
                    n2507 = Unbundle(w4513) -> ("CYCLE"=w4515:dbl)  [unwired: 2 out]
                    n2508 = stacked-sequence {
                      tunnel: w4520 -> [w4524 w4543]
                      tunnel: w4519 -> [_ w4542]
                      tunnel: w4518 -> [w4523 w4541]
                      tunnel: w4517 -> [w4522 w4540]
                      tunnel: w4516 -> [_ w4539]
                      tunnel: w4515 -> [_ w4538]
                      tunnel: w4512 -> [_ w4537]
                      tunnel: w4511 -> [w4525 _]
                      tunnel: w4510 -> [w4521 w4535]
                      tunnel: w4509 -> [_ w4536]
                      tunnel: w4508 -> [_ w4531]
                      frame #0 {
                        n2509 = case shown="True" w4525 {
                          tunnel: w4524 -> [_ w4530]
                          tunnel: w4523 -> [_ w4529]
                          tunnel: w4522 -> [_ w4528]
                          tunnel: w4521 -> [_ w4526]
                          frame False {
                          }
                          frame True {
                            n2510 = Bundle(cluster=w4526, "amps"=w4530, "volts"=w4529, "pf"=w4528) -> (w4527:cluster{"amps":dbl, "volts":dbl, "pf":dbl})
                            n2511 = local write "ON L03-2"(w4527) -> ()
                          }
                        }
                      }
                      frame #1 {
                        n2512 = Unbundle(w4535) -> ("amps"=w4534:dbl, "volts"=w4533:dbl, "pf"=w4532:dbl)
                        n2513 = case shown="True" w4536 {
                          tunnel: w4543 -> [_ w4575]
                          tunnel: w4542 -> [_ w4582]
                          tunnel: w4541 -> [_ _]
                          tunnel: w4540 -> [_ _]
                          tunnel: w4539 -> [_ w4581]
                          tunnel: w4538 -> [_ w4580]
                          tunnel: w4537 -> [_ w4545]
                          tunnel: w4534 -> [_ w4577]
                          tunnel: w4533 -> [_ w4576]
                          tunnel: w4532 -> [_ w4574]
                          tunnel: w4531 -> [_ w4566]
                          frame False {
                          }
                          frame True {
                            n2514 = local read "TDMS LAB03-2"() -> (w4579:refnum<k34>)
                            n2515 = Build Array(w4576) -> (w4571:dbl[])
                            n2516 = Build Array(w4574) -> (w4570:dbl[])
                            n2517 = Build Array(w4581) -> (w4569:dbl[])
                            n2518 = Build Array(w4582) -> (w4568:dbl[])
                            n2519 = Build Array(w4577) -> (w4573:dbl[])
                            n2520 = Build Array(w4575) -> (w4572:dbl[])
                            n2521 = Build Array(w4580) -> (w4567:dbl[])
                            n2522 = Build Array("AMPS ON", "AMPS OFF", "VOLTS", "PF", "TEMP Live", "TEMP Neut", "CYCLE") -> (w4550:string[])
                            n2523 = Bundle By Name("Y"=w4573, "t0"=w4566) -> (w4565:waveform(dbl))  [unwired: 1 in]
                            n2524 = Bundle By Name("Y"=w4572, "t0"=w4566) -> (w4564:waveform(dbl))  [unwired: 1 in]
                            n2525 = Bundle By Name("Y"=w4571, "t0"=w4566) -> (w4563:waveform(dbl))  [unwired: 1 in]
                            n2526 = Bundle By Name("Y"=w4570, "t0"=w4566) -> (w4562:waveform(dbl))  [unwired: 1 in]
                            n2527 = Bundle By Name("Y"=w4569, "t0"=w4566) -> (w4561:waveform(dbl))  [unwired: 1 in]
                            n2528 = Bundle By Name("Y"=w4568, "t0"=w4566) -> (w4560:waveform(dbl))  [unwired: 1 in]
                            n2529 = Bundle By Name("Y"=w4567, "t0"=w4566) -> (w4559:waveform(dbl))  [unwired: 1 in]
                            n2530 = Build Array(w4565, w4564, w4563, w4562, w4561, w4560, w4559) -> (w4558:waveform(dbl)[])
                            n2531 = TDMS Write(0:w4579, 5:"TEST VALUES", 7:w4550, 9:w4558) -> (4:w4549:refnum<k34>, 6:w4548:string, 15:w4547:errorcluster)  [unwired: 2 in, 1 out]
                            n2532 = TDMS Write(0:w4549, 5:w4548, 7:"TIME", 9:w4545, 11:w4547) -> (15:w4544:errorcluster)  [unwired: 1 in, 3 out]
                            n2533 = local write "data file error"(w4544) -> ()
                          }
                        }
                      }
                    }
                  }
                }
              }
              frame #6 {
